vi "NI VeriStand - Send Custom Device Message.vi"   [LabVIEW 2020, in "NI_VS Custom Device ExecutionAPI.lvlib"]
doc: "Sends a message or command to a custom device in an NI VeriStand project, as well as data required by the case that handles the command. You can use this VI with any custom device that registers to receive the <B>Command</B> you specify."
uses:
  <vilib>/NI VeriStand/Execution/CustomDevice/NI_VS Custom Device ExecutionAPI.lvlib
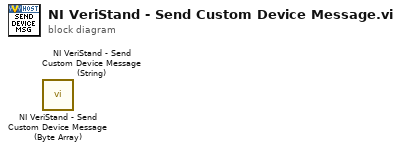
[diagram p0: block diagram]
diagram:
  n1 = call <vilib>:"NI VeriStand - Send Custom Device Message (Byte Array).vi"() -> ()  [unwired: 9 in, 3 out]
  n2 = call <vilib>:"NI VeriStand - Send Custom Device Message (String).vi"() -> ()  [unwired: 9 in, 3 out]
